vi "Board Size.vi"(11 "Square in":refnum<class "Square.lvclass">) -> (2 "Board Size":i16)   [LabVIEW 2020, in "SquareBattle.lvlib" / "Square.lvclass"]
uses:
  Square.lvclass
  Square.lvclass/Square.ctl
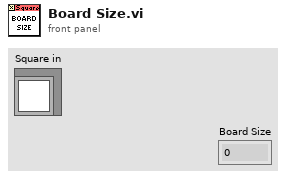
[diagram p1: front panel]
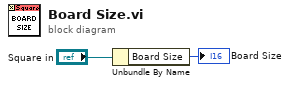
[diagram p0: block diagram]
diagram:
  n1 = Unbundle By Name("Square in") -> ("Board Size"=→"Board Size":i32)
